vi "TransformPoint.vi"(2 "P":T1={"X"=1.0, "Y"=0.0, "Z"=0.0, "w"=0.0} {"w" format="%.2f"; "Z" format="%.2f"; "Y" format="%.2f"; "X" format="%.2f"}, 3 "A":T2={"nx"=1.0, "ny"=0.0, "nz"=0.0, "nw"=0.0, "ox"=0.0, "oy"=1.0, "oz"=0.0, "ow"=0.0, "ax"=0.0, "ay"=0.0, "az"=1.0, "aw"=0.0, "Px"=5.0, "Py"=2.0, "Pz"=3.0, "Pw"=1.0} {"Pw" format="%.2f"; "Pz" format="%.2f"; "Py" format="%.2f"; "Px" format="%.2f"; "aw" format="%.2f"; "az" format="%.2f"; "ay" format="%.2f"; "ax" format="%.2f"; "ow" format="%.2f"; "nw" format="%.2f"; "oz" format="%.2f"; "oy" format="%.2f"; "ox" format="%.2f"; "nz" format="%.2f"; "ny" format="%.2f"; "nx" format="%.2f"}) -> (0 "error":i32, 1 "AxP":T1={"X"=1.0, "Y"=0.0, "Z"=0.0, "w"=0.0} {"w" format="%.2f"; "Z" format="%.2f"; "Y" format="%.2f"; "X" format="%.2f"})   [LabVIEW 2010]
uses:
  <vilib>/Analysis/NI_AALBase.lvlib
  <vilib>/Analysis/baseanly.llb/A x Vector.vi
  ReferenceFrame.ctl
  SinglePoint.ctl
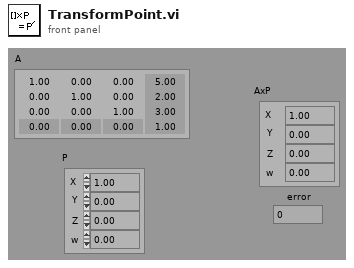
[diagram p1: front panel]
types:
  T1 = typedef "SinglePoint.ctl" = cluster{"X":dbl, "Y":dbl, "Z":dbl, "w":dbl}
  T2 = typedef "ReferenceFrame.ctl" = cluster{"nx":dbl, "ny":dbl, "nz":dbl, "nw":dbl, "ox":dbl, "oy":dbl, "oz":dbl, "ow":dbl, "ax":dbl, "ay":dbl, "az":dbl, "aw":dbl, "Px":dbl, "Py":dbl, "Pz":dbl, "Pw":dbl}
  T3 = cluster{"A x Vector[0]":dbl, "A x Vector[1]":dbl, "A x Vector[2]":dbl, "A x Vector[3]":dbl}
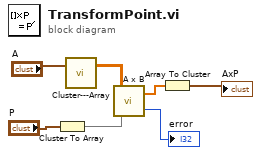
[diagram p0: block diagram]
diagram:
  n1 = Cluster To Array(cluster="P") -> (array=w3:dbl[])
  n2 = call "Cluster---Array.vi"("A"="A") -> ("Array (A)"=w6:dbl[][])  [unwired: 1 in, 1 out]
  n3 = call-poly <vilib>:"A x B.vi"("Vector"=w3, "A"=w6) -> ("error"=→"error":i32, "A x Vector"=w2:dbl[])
  n4 = Array To Cluster(array=w2) -> (cluster=→"AxP":T3)
